vi "ESP32_Socket_Example.vi"() -> ()   [LabVIEW 2022 SP3]
doc: "Demonstrates how to open a connection to an TCP server, read the data being sent, and display the data on a chart. This VI is designed to stop if the TCP connection is terminated."
panel:
  out "Numeric":i32
  out "data out":string
  in  "address":string="10.0.0.127"
  in  "Server Closed":string="The server VI closed the connection."
  in  "Stop":bool
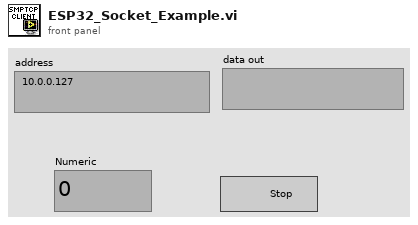
[diagram p1: front panel]
types:
  T1 = enum16{"Standard", "Buffered", "CRLF", "Immediate"}
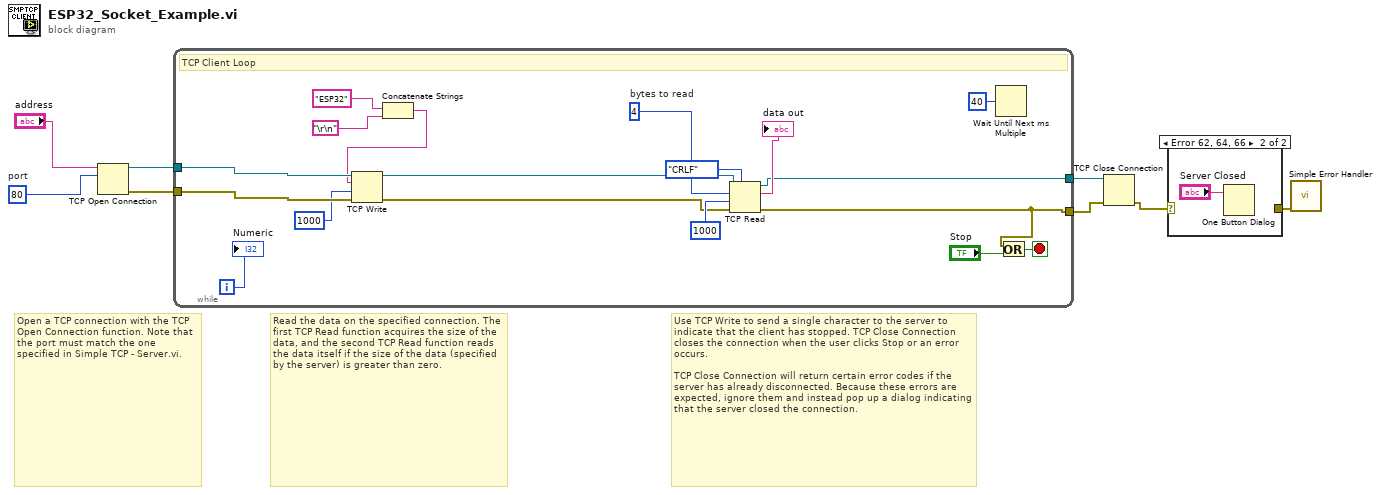
[diagram p0: block diagram]
diagram:
  w4 = u16 80  # port
  # "Use TCP Write to send a single character to the server to indicate that the client has stopped. TCP Close Connection closes the connection when the user clicks Stop or an error occurs.\n\nTCP Close Connection will return certain error codes if the server has already disconnected. Because these errors are expected, ignore them and instead pop up a dialog indicating that the server closed the connection."
  # "Read the data on the specified connection. The first TCP Read function acquires the size of the data, and the second TCP Read function reads the data itself if the size of the data (specified by the server) is greater than zero."
  # "Open a TCP connection with the TCP Open Connection function. Note that the port must match the one specified in Simple TCP - Server.vi."
  n1 = TCP Open Connection(address="address", remote port or service name=w4) -> (connection ID=w2:refnum<k5>, error out=w1:errorcluster)  [unwired: 3 in]
  n2 = while {
    tunnel: [w16] -> w7
    tunnel: [w17] -> w6
    tunnel: w2 -> [w15]
    tunnel: w1 -> [w14]
    i -> [w18]
    stop <- w24 stop-if-true
    w26 = 4  # bytes to read
    # "TCP Client Loop"
    n3 = Concatenate Strings("ESP32" ("data in"), "\r\n") -> (w10:string)
    n4 = TCP Write(connection ID=w15, data in=w10, error in (no error)=w14, 9:1000 ("timeout ms (25000)")) -> (connection ID out=w21:refnum<k5>, error out=w9:errorcluster)  [unwired: 1 out]
    n5 = TCP Read(connection ID=w21, bytes to read=w26, error in (no error)=w9, 7:T1."CRLF" ("mode (standard)"), 9:1000 ("timeout ms (25000)")) -> (connection ID out=w17:refnum<k5>, data out=→"data out":string, error out=w16:errorcluster)
    n6 = Wait Until Next ms Multiple(millisecond multiple=u32 40) -> ()  [unwired: 1 out]
    n7 = Or(x=w16, y="Stop") -> (x .or. y?=w24:bool)
    "Numeric" <- w18
  }
  n8 = TCP Close Connection(connection ID=w6, error in (no error)=w7) -> (error out=w5:errorcluster)  [unwired: 1 in, 1 out]
  n9 = case shown="Error 62, 64, 66" w5 {
    selector: w5 -> [w27 _]
    tunnel: [w27 _] -> w8
    frame #0 {
    }
    frame #1 {
      n10 = One Button Dialog(message="Server Closed") -> ()  [unwired: 1 in, 1 out]
    }
  }
  n11 = call <vilib>:"Simple Error Handler.vi"("error in (no error)"=w8) -> ()  [unwired: 4 in, 5 out]
